vi "move.vi"(1 "v":dbl=10.0, 2 "n":i32=1, 3 "String":string(combo)="home", 4 "z":dbl, 5 "y":dbl, 6 "x":dbl, 7 "连接ID":refnum<k5>) -> (0 "连接ID输出":refnum<k5>)   [LabVIEW 2017]
uses:
  <vilib>/LVH/i3 JSON/JSON Generation/Add Object Parameter Files/Add Object Parameter - Numeric.vi
  <vilib>/LVH/i3 JSON/i3-json.lvlib
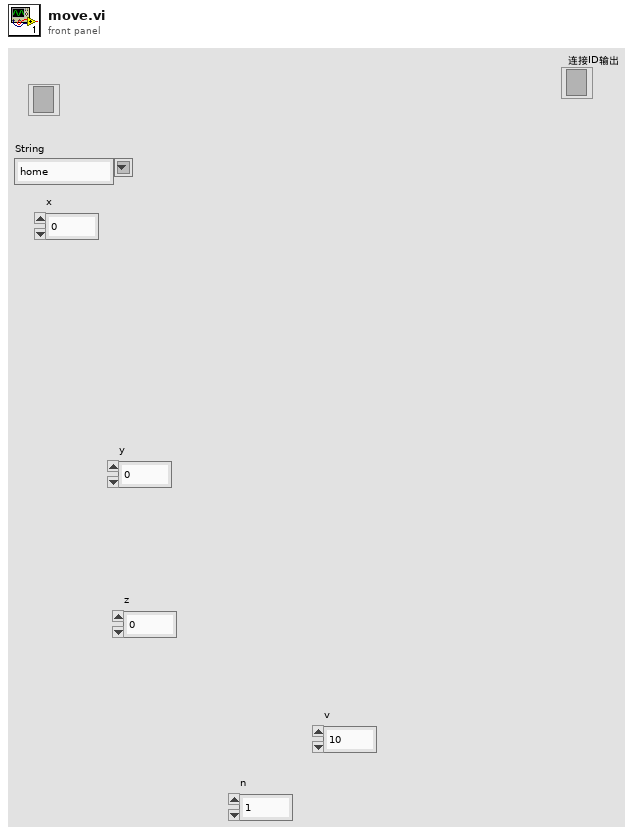
[diagram p1: front panel]
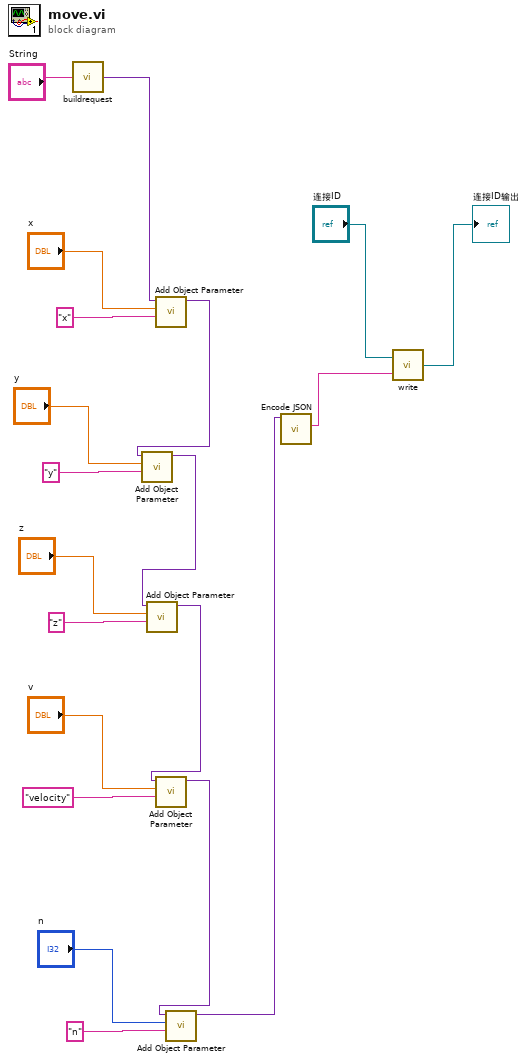
[diagram p0: block diagram]
diagram:
  n1 = call "buildrequest.vi"("String"="String") -> ("JSON Tree out (JSON Object)"=w8:variant)
  n2 = call-poly <vilib>:"Add Object Parameter.vi"("Name"="x", "Numeric"="x", "JSON Tree in (JSON Object)"=w8) -> ("JSON Tree out (JSON Object)"=w7:variant)  [unwired: 7 in, 1 out]
  n3 = call-poly <vilib>:"Add Object Parameter.vi"("Name"="y", "Numeric"="y", "JSON Tree in (JSON Object)"=w7) -> ("JSON Tree out (JSON Object)"=w6:variant)  [unwired: 7 in, 1 out]
  n4 = call-poly <vilib>:"Add Object Parameter.vi"("Name"="z", "Numeric"="z", "JSON Tree in (JSON Object)"=w6) -> ("JSON Tree out (JSON Object)"=w5:variant)  [unwired: 7 in, 1 out]
  n5 = call-poly <vilib>:"Add Object Parameter.vi"("Name"="velocity", "Numeric"="v", "JSON Tree in (JSON Object)"=w5) -> ("JSON Tree out (JSON Object)"=w2:variant)  [unwired: 7 in, 1 out]
  n6 = call-poly <vilib>:"Add Object Parameter.vi"("Name"="n", "Numeric"="n", "JSON Tree in (JSON Object)"=w2) -> ("JSON Tree out (JSON Object)"=w1:variant)  [unwired: 7 in, 1 out]
  n7 = call <vilib>:"Encode JSON.vi"("JSON Tree"=w1) -> ("String"=w20:string)  [unwired: 5 in, 1 out]
  n8 = call "write.vi"("数据输入"=w20, "连接ID"="连接ID") -> ("连接ID输出"=→"连接ID输出":refnum<k5>)
